vi "Lift Controller.vi"(8 "error in":errorcluster) -> ()   [LabVIEW 2019]
doc: "This VI executes continuously carrying out the current operation and responding to updates or new operations. It will often contain the timing or control code that is difficult to place directly in TeleOp. This VI generally opens all sensors and motors and isolates the rest of the robot code from knowing how the operations are carried out."
uses:
  <vilib>/Rock Robotics/WPI/Framework/Completion Status.ctl
  Lift Setpoints.ctl
  Lift Operations.ctl
  <vilib>/Rock Robotics/WPI/ThirdParty/Phoenix-LabVIEW/Motor Controller/Controls/CTRE_Phoenix_MotorControl_ControlMode.ctl
  <vilib>/Rock Robotics/Network Tables/NT Write Boolean.vi
panel:
  in  "Interactive Values":T1
  out "Current\nCmd":string
  in  "Buttons":cluster{"Execute Cmd":bool, "Abort Cmd":bool}
  out "Command Timing":cluster{"Start Time (ms)":u32, "Iterations":i32}
  out "Status":T3
  # "Tip: It may be helpful to observe inputs and sensor values.\nYou may also want to display tuning or debugging controls."
  # "Interactive Command: You may fill in the settings for a command\nand schedule it with the Execute button. You can observe and abort\nany command while fine tuning the code for the controller."
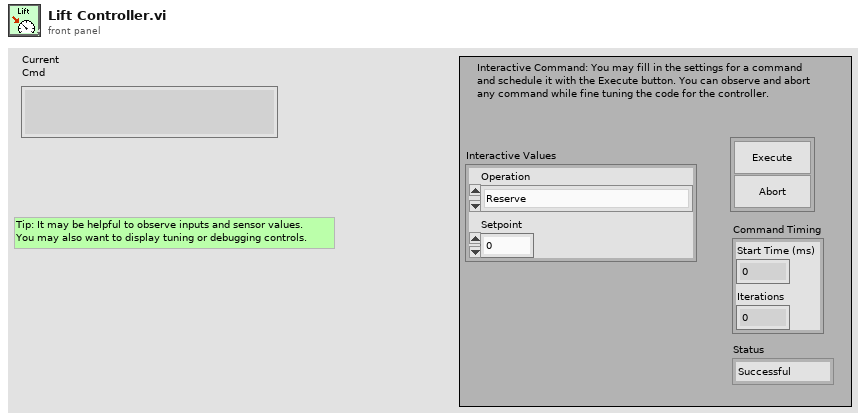
[diagram p1: front panel]
types:
  T1 = typedef "Lift Setpoints.ctl" = cluster{"Operation":T2, "Setpoint":dbl}
  T2 = typedef "Lift Operations.ctl" = enum16{"Reserve", "Read Current", "Immediate", "Lift"}
  T3 = typedef "Completion Status.ctl" = enum16{"Successful", "Aborted", "Incomplete"}
  T4 = enum16{"FollowerType_PercentOutput", "FollowerType_AuxOutput1"}
  T5 = typedef "WPI_MotorControlDeviceRef.ctl" = cluster{"DeviceStatus":errorcluster, "Type":T6, "PWM":cluster{"PWM Channel":T7, "DeadBand":T8}, "CAN":cluster{"Device Number":u8, "SetOutput VI Ref":variant, "GetOutput VI Ref":variant, "Enable VI Ref":variant, "Disable VI Ref":variant, "Data":variant}, "Invert":bool, "DIO PWM":cluster{"PWM \"Enable\" Channel":T7, "DIOChannel":T9, "PWM Rate":dbl}}
  T6 = typedef "WPI_MotorControlType.ctl" = enum16{"PWM", "CAN", "DIO PWM"}
  T7 = typedef "FPGA_DIOPWMChannel.ctl" = enum8{"PWM 0", "PWM 1", "PWM 2", "PWM 3", "PWM 4", "PWM 5", "PWM 6", "PWM 7", "PWM 8", "PWM 9", "PWM MXP 0", "PWM MXP 1", "PWM MXP 2", "PWM MXP 3", "PWM MXP 4", "PWM MXP 5", "PWM MXP 6", "PWM MXP 7", "PWM MXP 8", "PWM MXP 9", "Invalid"}
  T8 = typedef "WPI_PWMDeadband.ctl" = cluster{"Name":string, "maxPositivePwm":i32, "minPositivePwm":i32, "centerPwm":i32, "maxNegativePwm":i32, "minNegativePwm":i32, "angularRange":u16}
  T9 = typedef "FPGA_DIOChannel.ctl" = enum8{"DIO 0", "DIO 1", "DIO 2", "DIO 3", "DIO 4", "DIO 5", "DIO 6", "DIO 7", "DIO 8", "DIO 9", "DIO MXP 0", "DIO MXP 1", "DIO MXP 2", "DIO MXP 3", "DIO MXP 4", "DIO MXP 5", "DIO MXP 6", "DIO MXP 7", "DIO MXP 8", "DIO MXP 9", "DIO MXP 10", "DIO MXP 11", "DIO MXP 12", "DIO MXP 13", "DIO MXP 14", "DIO MXP 15", "SPI Port CS1", "SPI Port CS2", "SPI Port CS3", "SPI Port MISO", "SPI Port MOSI", "Invalid"}
  T10 = typedef "Command Status Info.ctl" = cluster{"Name":string, "Status":T3, "notifier out":T11}
  T11 = typedef "Completion Notifier.ctl" = refnum<notifier>
  T12 = cluster{"Current Command":T1, "Command Timing":cluster{"Start Time (ms)":u32, "Iterations":i32}, "Command Arguments":cluster{"Command Info":T10, "Description":string, "Default Command":T1, "queue out":refnum<queue>, "Subsystem Name":string}}
  T13 = typedef "CTRE_Phoenix_MotorControl_ControlMode.ctl" = u16
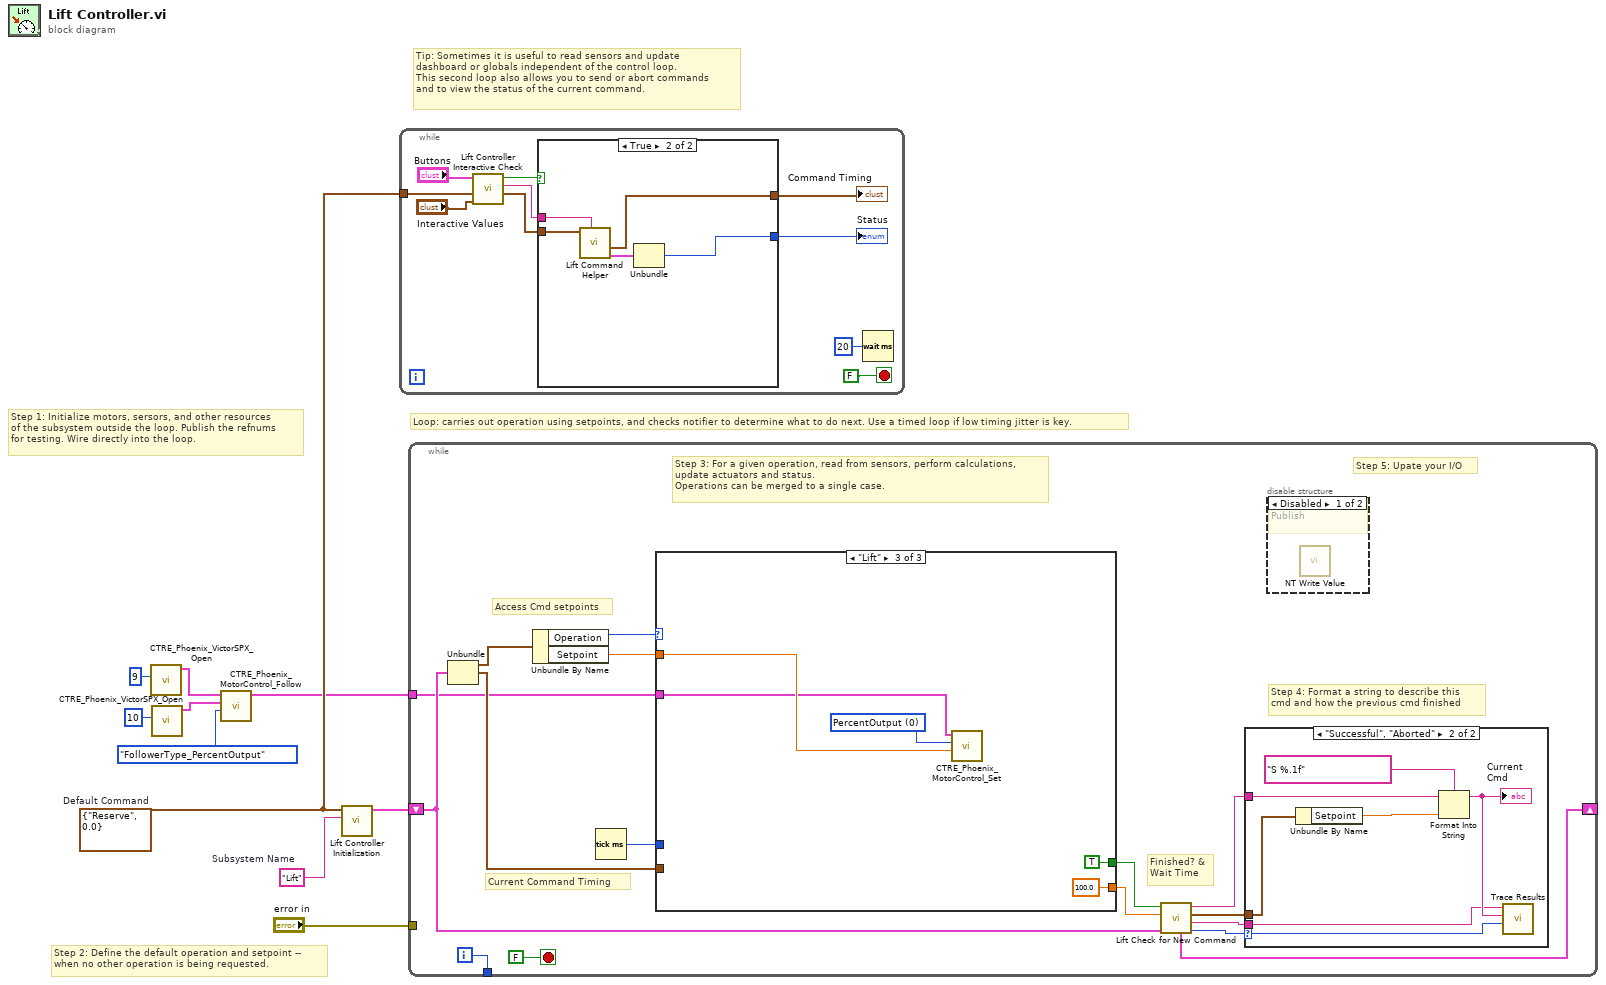
[diagram p0: block diagram]
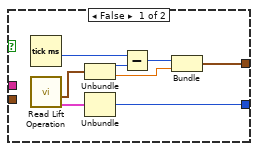
[diagram p2: hidden frame]
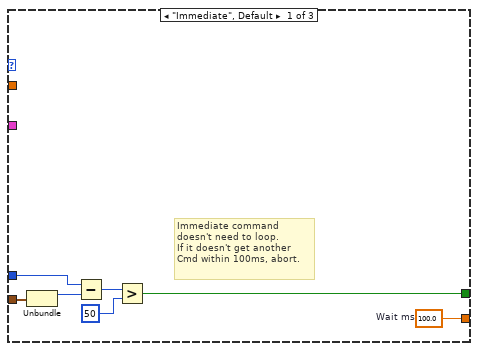
[diagram p5: hidden frame]
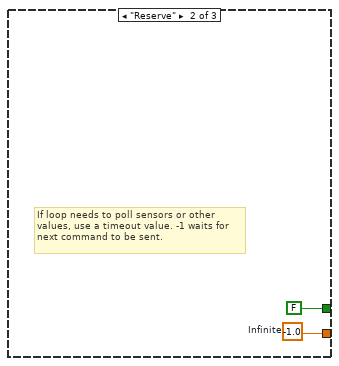
[diagram p6: hidden frame]
diagram:
  w7 = T1 {"Operation"=enum."Reserve", "Setpoint"=0.0}  # Default Command
  w8 = "Lift"  # Subsystem Name
  # "Tip: Sometimes it is useful to read sensors and update\ndashboard or globals independent of the control loop.\nThis second loop also allows you to send or abort commands\nand to view the status of the current command."
  # "Step 2: Define the default operation and setpoint --\nwhen no other operation is being requested."
  # "Step 1: Initialize motors, sersors, and other resources\nof the subsystem outside the loop. Publish the refnums\nfor testing. Wire directly into the loop."
  # "Loop: carries out operation using setpoints, and checks notifier to determine what to do next. Use a timed loop if low timing jitter is key."
  n1 = call <vilib>:"CTRE_Phoenix_VictorSPX_Open.vi"("Device Number"=u8 9) -> ("CAN Talon SRX Ref"=w4:T5)  [unwired: 9 in, 1 out]
  n2 = call <vilib>:"CTRE_Phoenix_VictorSPX_Open.vi"("Device Number"=u8 10) -> ("CAN Talon SRX Ref"=w3:T5)  [unwired: 9 in, 1 out]
  n3 = call <vilib>:"CTRE_Phoenix_MotorControl_Follow.vi"("FollowerType"=T4."FollowerType_PercentOutput", "Master Controller to Follow"=w3, "PhoenixMotorControlDevRef"=w4) -> ("PhoenixMotorControlDevRef"=w1:T5)  [unwired: 7 in, 1 out]
  n4 = call "Lift Controller Initialization.vi"("Subsystem Name"=w8, "Default Command"=w7) -> ("Current Command"=w9:T12)  [unwired: 9 in]
  n5 = while {
    tunnel: w7 -> [w17]
    stop <- FALSE stop-if-true
    n6 = call "Lift Controller Interactive Check.vi"("Interactive Command in"="Interactive Values", "Default Command"=w17, "Buttons"="Buttons") -> ("Interactive Command out"=w14:T1, "Trace String"=w15:string, "Schedule"=w16:bool)  [unwired: 6 in]
    n7 = case shown="True" w16 {
      tunnel: [w28 w33] -> w13
      tunnel: w14 -> [_ w31]
      tunnel: [w24 w29] -> w12
      tunnel: w15 -> [_ w32]
      frame False {
        n8 = Tick Count (ms)() -> (millisecond timer value=w23:u32)
        n9 = call "Read Lift Operation.vi"() -> ("Command Info"=w21:T10, "SubSystem Data"=w22:T1)  [unwired: 9 in, 1 out]
        n10 = Unbundle(w22) -> ("Operation"=w27:T2, "Setpoint"=w25:dbl)
        n11 = Unbundle(w21) -> ("Status"=w28:T3)  [unwired: 2 out]
        n12 = Subtract(x=w23, y=w27) -> (x-y=w26:u32)
        n13 = Bundle(w26, "Setpoint"=w25) -> (w24:cluster{u32, "Setpoint":dbl})  [unwired: 1 in]
      }
      frame True {
        n14 = call "Lift Command Helper.vi"("Description"=w32, "SubSystem Data"=w31) -> ("Command Info Out"=w30:T10, "Command Timing"=w29:cluster{"Start Time (ms)":u32, "Iterations":i32})  [unwired: 7 in, 1 out]
        n15 = Unbundle(w30) -> ("Status"=w33:T3)  [unwired: 2 out]
      }
    }
    "Status" <- w13
    "Command Timing" <- w12
    n16 = Wait (ms)(milliseconds to wait=u32 20) -> ()  [unwired: 1 out]
  }
  n17 = while {
    shift-right: [w43] -> _
    shift-left: w9 -> [w36]
    tunnel: [w48] -> _
    tunnel: "error in" -> [_]
    tunnel: w1 -> [w34]
    i -> [w48]
    stop <- FALSE stop-if-true
    # "Step 5: Upate your I/O"
    # "Step 4: Format a string to describe this\ncmd and how the previous cmd finished"
    # "Current Command Timing"
    # "Access Cmd setpoints"
    # "Finished? &\nWait Time"
    # "Step 3: For a given operation, read from sensors, perform calculations,\nupdate actuators and status.\nOperations can be merged to a single case."
    n18 = Unbundle(w36) -> ("Current Command"=w47:T1, "Command Timing"=w44:cluster{"Start Time (ms)":u32, "Iterations":i32})  [unwired: 1 out]
    n19 = Unbundle By Name(w47) -> ("Operation"=w46:T2, "Setpoint"=w35:dbl)
    n20 = Tick Count (ms)() -> (millisecond timer value=w45:u32)
    n21 = case shown="\"Lift\"" w46 {
      tunnel: [w63 w65 100.0 ("Infinite")] -> w41
      tunnel: [w57 FALSE ("ignore previous (F)") TRUE ("ignore previous (F)")] -> w42
      tunnel: w44 -> [w59 _ _]
      tunnel: w45 -> [w58 _ _]
      tunnel: w35 -> [_ _ w67]
      tunnel: w34 -> [_ _ w66]
      frame "Immediate", Default {
        w63 = 100.0  # Wait ms
        # "Immediate command\ndoesn't need to loop.\nIf it doesn't get another\nCmd within 100ms, abort."
        n22 = Unbundle(w59) -> ("Start Time (ms)"=w62:u32)  [unwired: 1 out]
        n23 = Subtract(x=w58, y=w62) -> (x-y=w61:u32)
        n24 = Greater?(x=w61, y=u8 50 ("Left Motor")) -> (0:w57:bool)
      }
      frame "Reserve" {
        w65 = -1.0  # Infinite
        # "If loop needs to poll sensors or other\nvalues, use a timeout value. -1 waits for\nnext command to be sent."
      }
      frame "Lift" {
        w70 = T13 0 items=["PercentOutput"=0, "Position"=1, "Velocity"=2, "Current"=3, "Follower"=5, "MotionProfile"=6, "MotionMagic"=7, "MotionProfileArc"=10, "Disabled"=15] ("Control Mode")
        n25 = call <vilib>:"CTRE_Phoenix_MotorControl_Set.vi"("Output"=w67, "Control Mode"=w70, "PhoenixMotorControlDevRef"=w66) -> ()  [unwired: 7 in, 2 out]
      }
    }
    n26 = call "Lift Check for New Command.vi"("Current Command"=w36, "Wait time (ms)"=w41, "Finished?"=w42) -> ("Completion"=w37:T3, "Subsystem Name"=w38:string, "Current Command"=w39:T1, "Initial Trace String"=w40:string, "NextCommand"=w43:T12)  [unwired: 4 in]
    n27 = case shown="\"Successful\", \"Aborted\"" w37 {
      selector: w37 -> [_ w56]
      tunnel: w40 -> [_ w52]
      tunnel: w39 -> [_ w53]
      tunnel: w38 -> [_ w50]
      frame "Incomplete", Default {
        # "Continuing current command"
      }
      frame "Successful", "Aborted" {
        # "Report and setup for next command"
        n28 = Unbundle By Name(w53) -> ("Setpoint"=w55:dbl)
        n29 = Format Into String(format string="S %.1f", initial string=w52, w55) -> (resulting string=w51:string)  [unwired: 1 in, 1 out]
        "Current\nCmd" <- w51
        n30 = call <vilib>:"Trace Results.vi"("Status of previous command"=w56, "Description"=w51, "Subsystem"=w50) -> ()  [unwired: 9 in]
      }
    }
    n31 = disable-structure shown="Disabled" {
      frame Disabled {
        # "Publish"
        n32 = call-poly <vilib>:"NT Write Value.vi"() -> ()  [unwired: 11 in, 1 out]
      }
      frame Enabled {
      }
    }
  }
